vi "Detailed View.vi"(8 "error in (no error)":errorcluster, 10 "Server URL":refnum<k21>="\\\\localhost\\ABCDEFG", 11 "Client Message Queues":T1) -> ()   [LabVIEW 2024]
doc: "This VI is a user interface VI of the client and is used to display the detailed information of a subsystem, including the graphic subsystem view, alarm & event view, and historical data view."
uses:
  Shared/Message Queue/Client Message Queues.ctl
  Shared/Message Queue/Message Cluster.ctl
  Controls/Client/Detailed View - Data.ctl
  Error Handlers/Error Message.ctl
  Shared/Message Queue.lvlib
  Shared/User Event - Stop.lvlib
panel:
  in  "Exit":bool
  in  "Refresh":bool
  in  "Alarm & Event List":bool
  in  "Subsystem":string(combo)
  in  "Historical Trend":bool
  in  "Subsystem View":bool
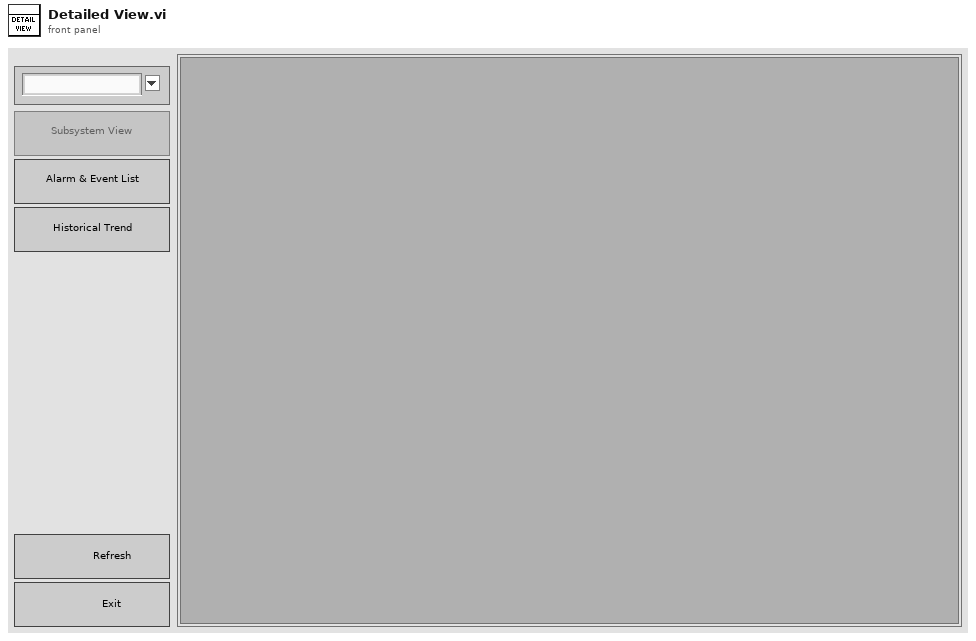
[diagram p1: front panel]
types:
  T1 = typedef "Message Queue.lvlib/Client Message Queues.ctl" = cluster{"Client Main":refnum<queue>, "Detailed View":refnum<queue>}
  T2 = typedef "Detailed View - Data.ctl" = cluster{"Current View Name":string, "Current View":refnum<vi>, "Current Subsystem":string, "Subview Reference Map":variant, "Subview Stop Events":refnum<user-event>[], "Detailed View Stop Event":refnum<user-event>, "Subview Switch Buttons Map":variant, "Client Message Queues":T1}
  T3 = typedef "Error Message.ctl" = cluster{"Error":errorcluster, "Component":string}
  T4 = enum8{"Enabled", "Disabled", "Disabled and Grayed Out"}
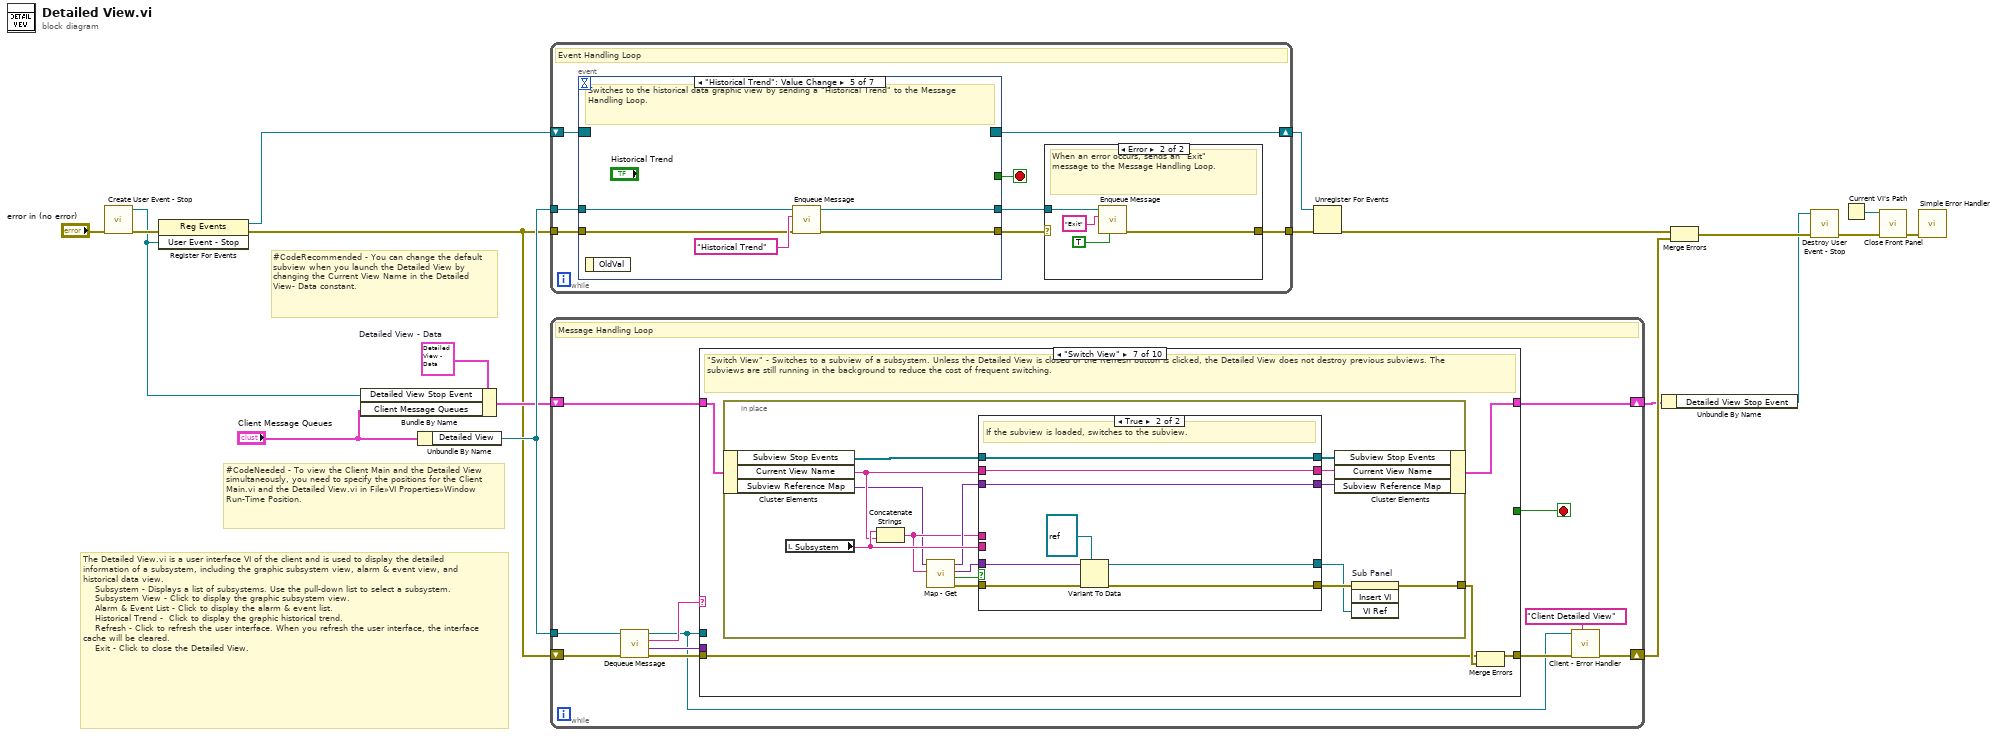
[diagram p0: block diagram]
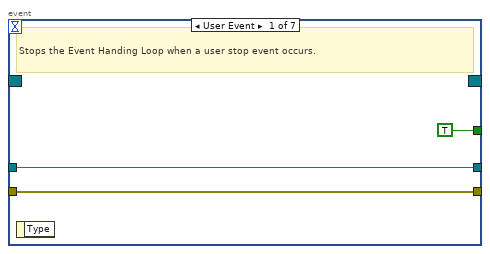
[diagram p3: hidden frame]
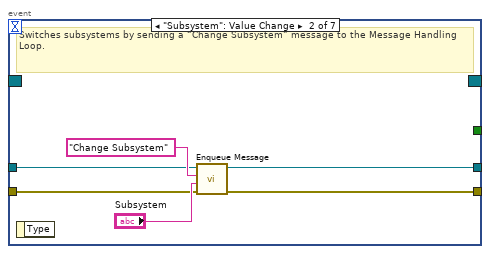
[diagram p4: hidden frame]
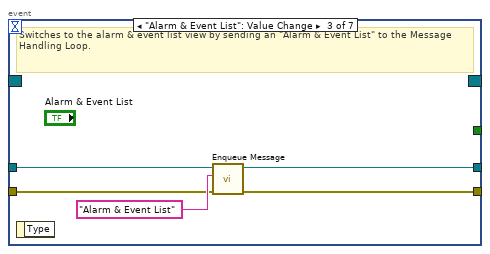
[diagram p5: hidden frame]
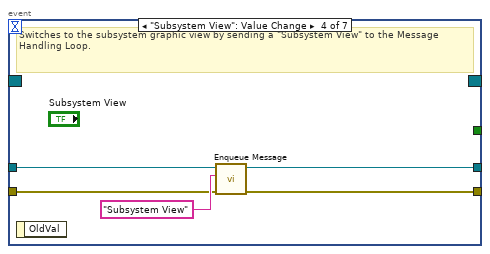
[diagram p6: hidden frame]
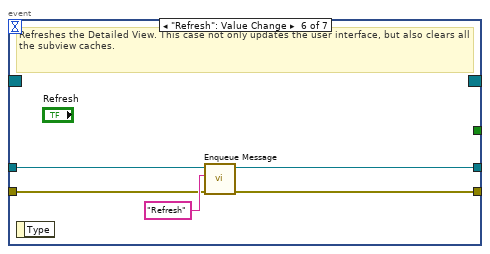
[diagram p7: hidden frame]
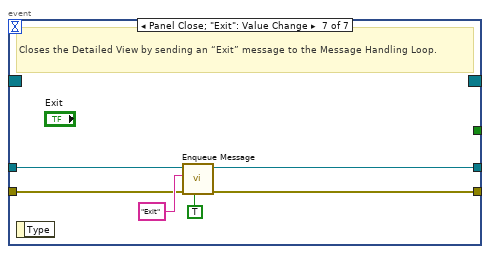
[diagram p8: hidden frame]
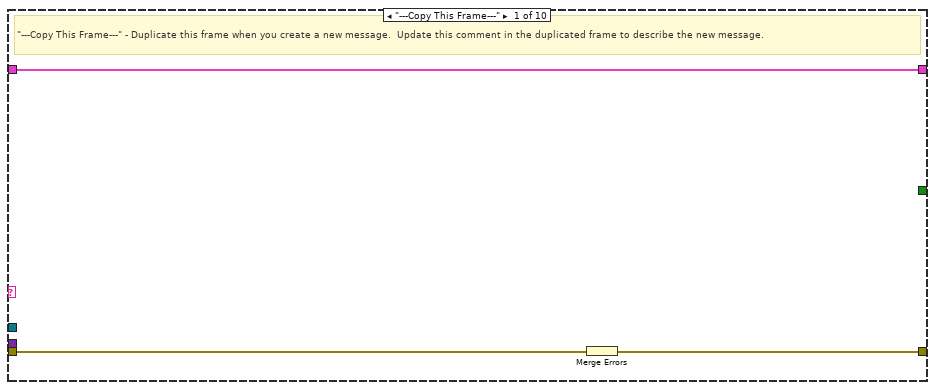
[diagram p9: hidden frame]
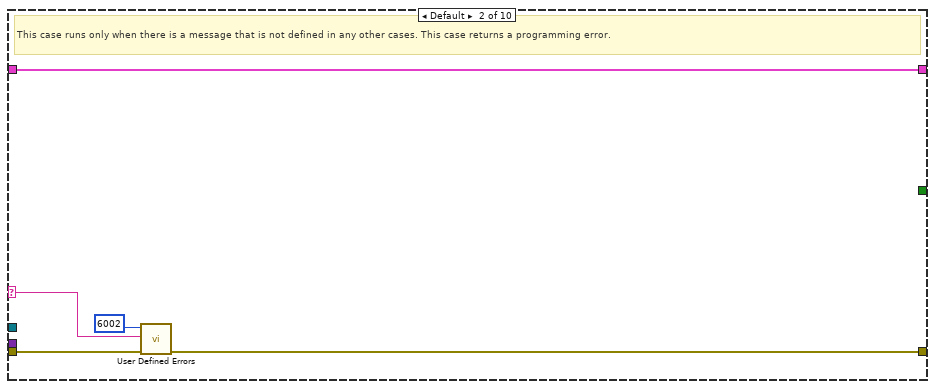
[diagram p10: hidden frame]
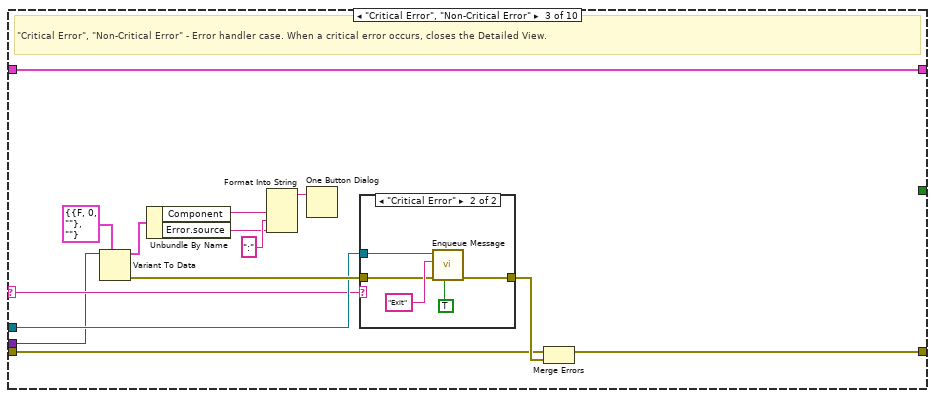
[diagram p11: hidden frame]
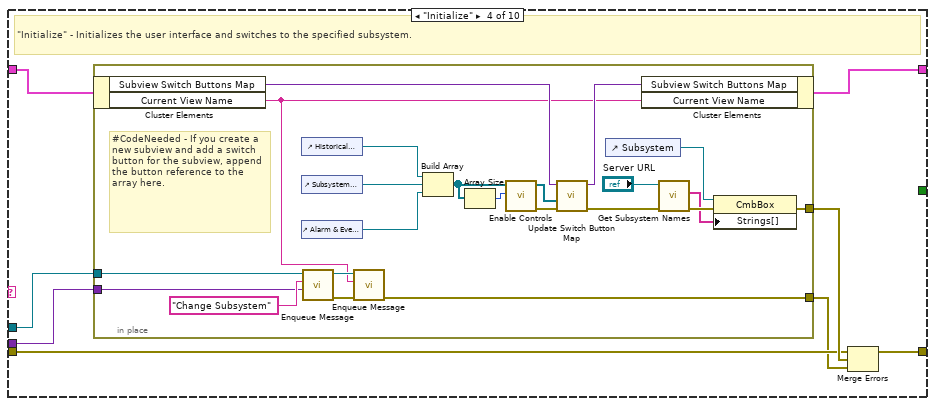
[diagram p13: hidden frame]
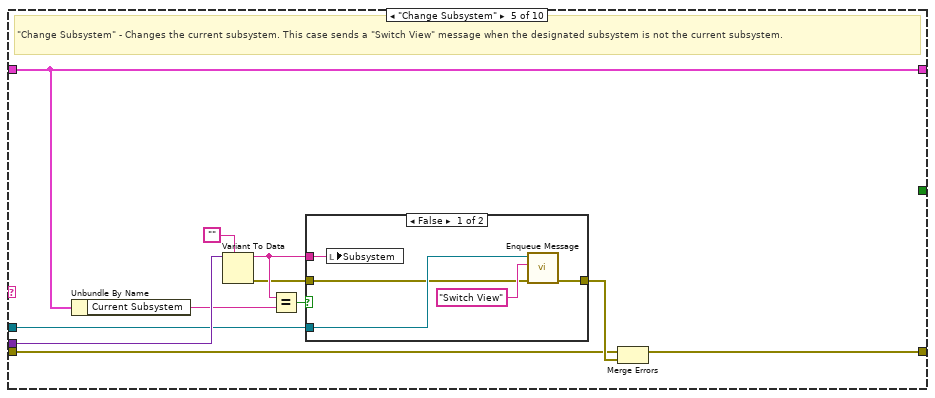
[diagram p14: hidden frame]
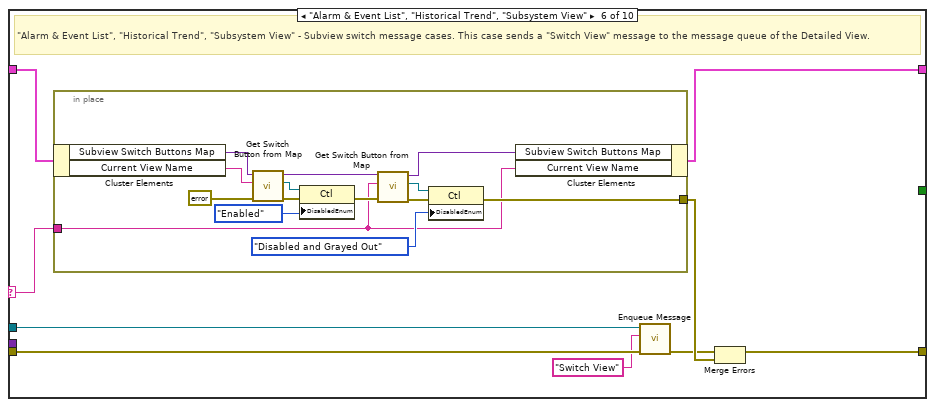
[diagram p16: hidden frame]
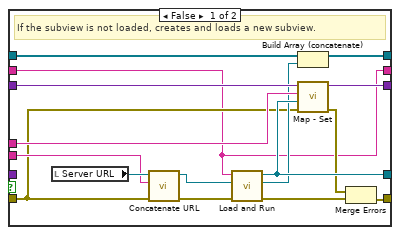
[diagram p17: hidden frame]
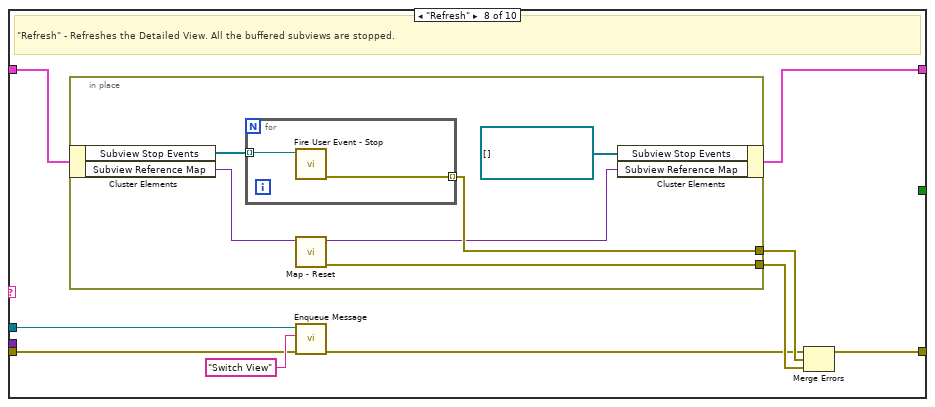
[diagram p18: hidden frame]
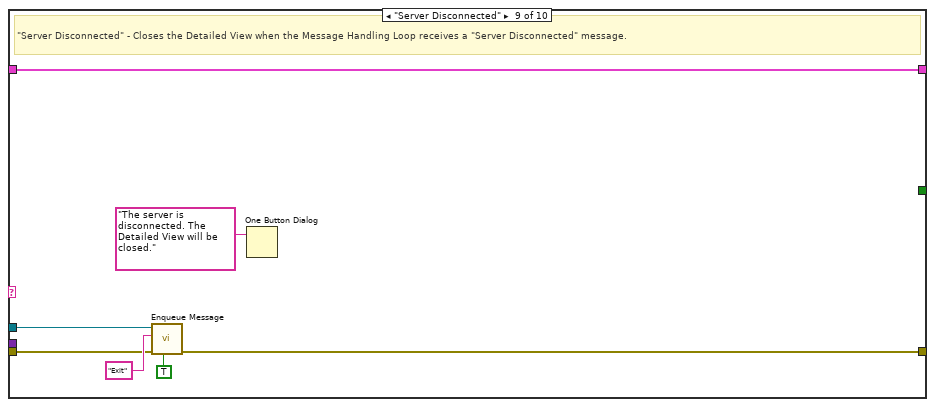
[diagram p19: hidden frame]
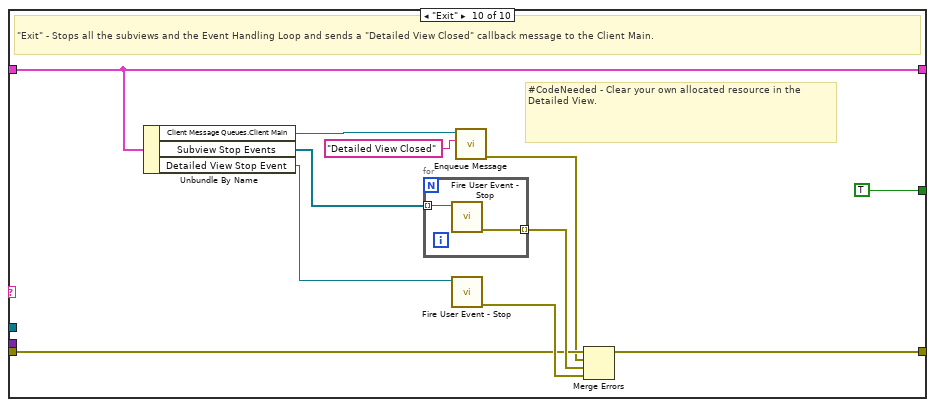
[diagram p20: hidden frame]
diagram:
  w12 = T2 {"Current View Name"="Subsystem View", "Current View"=refnum, "Current Subsystem"="", "Subview Reference Map"=variant, "Subview Stop Events"=[], "Detailed View Stop Event"=refnum, "Subview Switch Buttons Map"=variant, "Client Message Queues"={"Client Main"=refnum, "Detailed View"=refnum}}  # Detailed View - Data
  # "#CodeNeeded - To view the Client Main and the Detailed View simultaneously, you need to specify the positions for the Client Main.vi and the Detailed View.vi in File»VI Properties»Window Run-Time Position."
  # "#CodeRecommended - You can change the default subview when you launch the Detailed View by changing the Current View Name in the Detailed View- Data constant."
  # "The Detailed View.vi is a user interface VI of the client and is used to display the detailed information of a subsystem, including the graphic subsystem view, alarm & event view, and historical data view.\n    Subsystem - Displays a list of subsystems. Use the pull-down list to select a subsystem. \n    Subsystem View - Click to display the graphic subsystem view.\n    Alarm & Event List - Click to display the alarm & event list.\n    Historical Trend -  Click to display the graphic historical trend.\n    Refresh - Click to refresh the user interface. When you refresh the user interface, the interface cache will be cleared.\n    Exit - Click to close the Detailed View."
  n1 = call "Create User Event - Stop.vi"("error in (no error)"="error in (no error)") -> ("error out"=w4:errorcluster, "User Event - Stop"=w1:refnum<user-event>)  [unwired: 9 in]
  n2 = register-events(error in=w4, w1) -> (reference out=w2:refnum<event-registration>, error out=w3:errorcluster)  [unwired: 1 in]
  n3 = Bundle By Name(cluster=w12, "Detailed View Stop Event"=w1, "Client Message Queues"="Client Message Queues") -> (w6:T2)
  n4 = Unbundle By Name("Client Message Queues") -> ("Detailed View"=w13:refnum<queue>)
  n5 = while "Event Handling Loop" {
    tunnel: w13 -> [w27]
    tunnel: [w22] -> w16
    shift-right: [w23] -> w15
    shift-left: w2 -> [w24]
    tunnel: w3 -> [w20]
    stop <- w21 stop-if-true
    # "Event Handling Loop"
    n6 = event shown="[4] \"Historical Trend\": Value Change" {
      selector: w24 -> [_ _ _ _ _ _ _]
      dyn-events: [_ _ _ _ _ _ _] -> w23
      timeout: _ -> [_ _ _ _ _ _ _]
      tunnel: [TRUE ("Discard?") _ _ _ _ _ _] -> w21
      tunnel: w27 -> [w35 w40 w45 w50 w55 w61 w65]
      tunnel: [w33 w38 w43 w48 w53 w58 w63] -> w25
      tunnel: [w35 w39 w44 w49 w54 w60 w64] -> w26
      tunnel: w20 -> [w33 w36 w42 w47 w52 w57 w62]
      event User Event {
        # "Stops the Event Handing Loop when a user stop event occurs."
        n7 = event-data() -> ()  [unwired: 1 in, 1 out]
      }
      event "Subsystem": Value Change {
        # "Switches subsystems by sending a “Change Subsystem” message to the Message Handling Loop."
        n8 = event-data() -> ()  [unwired: 1 in, 1 out]
        n9 = call "Enqueue Message.vi"("error in (no error)"=w36, "Message Data"="Subsystem", "Message"="Change Subsystem", "Message Queue"=w40) -> ("error out"=w38:errorcluster, "dup Message Queue"=w39:refnum<queue>)  [unwired: 6 in]
      }
      event "Alarm & Event List": Value Change {
        # "Switches to the alarm & event list view by sending an \"Alarm & Event List\" to the Message Handling Loop."
        n10 = event-data() -> ()  [unwired: 1 in, 1 out]
        n11 = call "Enqueue Message.vi"("error in (no error)"=w42, "Message"="Alarm & Event List", "Message Queue"=w45) -> ("error out"=w43:errorcluster, "dup Message Queue"=w44:refnum<queue>)  [unwired: 7 in]
      }
      event "Subsystem View": Value Change {
        # "Switches to the subsystem graphic view by sending a \"Subsystem View\" to the Message Handling Loop."
        n12 = event-data() -> ()  [unwired: 1 in, 1 out]
        n13 = call "Enqueue Message.vi"("error in (no error)"=w47, "Message"="Subsystem View", "Message Queue"=w50) -> ("error out"=w48:errorcluster, "dup Message Queue"=w49:refnum<queue>)  [unwired: 7 in]
      }
      event "Historical Trend": Value Change {
        # "Switches to the historical data graphic view by sending a \"Historical Trend\" to the Message Handling Loop."
        n14 = event-data() -> ()  [unwired: 1 in, 1 out]
        n15 = call "Enqueue Message.vi"("error in (no error)"=w52, "Message"="Historical Trend", "Message Queue"=w55) -> ("error out"=w53:errorcluster, "dup Message Queue"=w54:refnum<queue>)  [unwired: 7 in]
      }
      event "Refresh": Value Change {
        # "Refreshes the Detailed View. This case not only updates the user interface, but also clears all the subview caches."
        n16 = event-data() -> ()  [unwired: 1 in, 1 out]
        n17 = call "Enqueue Message.vi"("error in (no error)"=w57, "Message"="Refresh", "Message Queue"=w61) -> ("error out"=w58:errorcluster, "dup Message Queue"=w60:refnum<queue>)  [unwired: 7 in]
      }
      event Panel Close; "Exit": Value Change {
        # "Closes the Detailed View by sending an “Exit” message to the Message Handling Loop."
        n18 = event-data() -> ()  [unwired: 1 in, 1 out]
        n19 = call "Enqueue Message.vi"("Priority Message? (F)"=TRUE, "error in (no error)"=w62, "Message"="Exit", "Message Queue"=w65) -> ("error out"=w63:errorcluster, "dup Message Queue"=w64:refnum<queue>)  [unwired: 6 in]
      }
    }
    n20 = case shown="Error" w25 {
      selector: w25 -> [w28 _]
      tunnel: w26 -> [_ w32]
      tunnel: [w28 w29] -> w22
      frame No Error {
      }
      frame Error {
        # "When an error occurs, sends an \"Exit\" message to the Message Handling Loop."
        n21 = call "Enqueue Message.vi"("Priority Message? (F)"=TRUE, "Message"="Exit", "Message Queue"=w32) -> ("error out"=w29:errorcluster)  [unwired: 7 in, 1 out]
      }
    }
  }
  n22 = while "Message Handling Loop" {
    tunnel: w13 -> [w72]
    shift-right: [w78] -> w11
    shift-left: w6 -> [w79]
    shift-right: [w70] -> w19
    shift-left: w3 -> [w76]
    stop <- w77 stop-if-true
    # "Message Handling Loop"
    n23 = call "Dequeue Message.vi"("error in (no error)"=w76, "Message Queue"=w72) -> ("error out"=w75:errorcluster, "Message Data"=w73:variant, "Message"=w74:string, "dup Message Queue"=w69:refnum<queue>)  [unwired: 6 in]
    n24 = case "Message Cases" shown="\"Switch View\"" w74 {
      selector: w74 -> [_ w84 w96 _ _ w157 _ _ _ _]
      tunnel: w69 -> [_ _ w97 w110 w144 w163 _ w227 w241 _]
      tunnel: w75 -> [w82 w83 w88 w113 w138 w162 w178 w228 w242 w249]
      tunnel: [w81 w85 w95 w115 w148 w160 w182 w230 w240 w255] -> w71
      tunnel: w79 -> [w80 w87 w101 w112 w142 w159 w179 w224 w245 w253]
      tunnel: [w80 w87 w101 w111 w142 w158 w180 w223 w245 w253] -> w78
      tunnel: [_ _ _ _ _ _ _ _ _ TRUE] -> w77
      tunnel: w73 -> [_ _ w94 w109 w147 _ _ _ _ _]
      frame "---Copy This Frame---" {
        # "\"---Copy This Frame---\" - Duplicate this frame when you create a new message.  Update this comment in the duplicated frame to describe the new message."
        n25 = Merge Errors(w82) -> (w81:errorcluster)
      }
      frame Default {
        # "This case runs only when there is a message that is not defined in any other cases. This case returns a programming error."
        n26 = call "User Defined Errors.vi"("error in (no error)"=w83, "Parameter 1"=w84, "Error Code (0)"=6002 ("error code (0)")) -> ("error out"=w85:errorcluster)  [unwired: 8 in]
      }
      frame "Critical Error", "Non-Critical Error" {
        # "\"Critical Error\", \"Non-Critical Error\" - Error handler case. When a critical error occurs, closes the Detailed View."
        n27 = Variant To Data(type=T3 {"Error"={"status"=FALSE, "code"=0, "source"=""}, "Component"=""} ("Error Message"), Variant=w94) -> (data=w100:T3, error out=w99:errorcluster)  [unwired: 1 in]
        n28 = Unbundle By Name(w100) -> ("Component"=w93:string, "Error.source"=w91:string)
        n29 = Format Into String(w93, ":" ("input 1"), w91) -> (resulting string=w90:string)  [unwired: 3 in, 1 out]
        n30 = One Button Dialog(message=w90) -> ()  [unwired: 1 in, 1 out]
        n31 = case shown="\"Critical Error\"" w96 {
          tunnel: [w102 w105] -> w89
          tunnel: w97 -> [_ w104]
          tunnel: w99 -> [w102 w103]
          frame Default {
          }
          frame "Critical Error" {
            n32 = call "Enqueue Message.vi"("Priority Message? (F)"=TRUE, "error in (no error)"=w103, "Message"="Exit", "Message Queue"=w104) -> ("error out"=w105:errorcluster)  [unwired: 6 in, 1 out]
          }
        }
        n33 = Merge Errors(w88, w89) -> (w95:errorcluster)
      }
      frame "Initialize" {
        # "\"Initialize\" - Initializes the user interface and switches to the specified subsystem."
        n34 = in-place {
          in-place-border: [w135] -> w114
          in-place-border: w110 -> [w119]
          in-place-border: w109 -> [w118]
          in-place-border: [w117] -> w108
          # "#CodeNeeded - If you create a new subview and add a switch button for the subview, append the button reference to the array here."
          n35 = in-place-cluster #1(w112) -> ("Subview Switch Buttons Map"=w124:variant, "Current View Name"=w116:string)
          n36 = control-ref of="Historical Trend"() -> (w134:refnum<vi>)
          n37 = control-ref of="Subsystem View"() -> (w133:refnum<vi>)
          n38 = control-ref of="Alarm & Event List"() -> (w131:refnum<vi>)
          n39 = call "Enqueue Message.vi"("Message Data"=w118, "Message"="Change Subsystem", "Message Queue"=w119) -> ("error out"=w122:errorcluster, "dup Message Queue"=w121:refnum<queue>)  [unwired: 7 in]
          n40 = call "Enqueue Message.vi"("error in (no error)"=w122, "Message"=w116, "Message Queue"=w121) -> ("error out"=w117:errorcluster)  [unwired: 7 in, 1 out]
          n41 = Build Array(w134, w133, w131) -> (w127:refnum<vi>[])
          n42 = Array Size(array=w127) -> (size(s)=w126:i32)
          n43 = call "Enable Controls.vi"("Number of Enabled Controls"=w126, "Controls"=w127) -> ("error out"=w129:errorcluster, "dup Controls"=w128:refnum<vi>[])  [unwired: 8 in]
          n44 = call "Update Switch Button Map.vi"("error in (no error)"=w129, "Binding Control Refnums"=w128, "URL Refnum Map In"=w124) -> ("error out"=w132:errorcluster, "URL Refnum Map Out"=w123:variant)  [unwired: 7 in]
          n45 = control-ref of="Subsystem"() -> (w130:refnum<vi>)
          n46 = in-place-cluster #1("Subview Switch Buttons Map"=w123, "Current View Name"=w116) -> (w111:T2)
          n47 = call "Get Subsystem Names.vi"("error in (no error)"=w132, "Server URL"="Server URL") -> ("error out"=w137:errorcluster, "Subsystem Names"=w125:string[])  [unwired: 7 in, 1 out]
          n48 = property class="CmbBox"(reference=w130, error in=w137, "Strings[]"=w125) -> (error out=w135:errorcluster)  [unwired: 1 out]
        }
        n49 = Merge Errors(w113, w114, w108) -> (w115:errorcluster)
      }
      frame "Change Subsystem" {
        # "\"Change Subsystem\" - Changes the current subsystem. This case sends a \"Switch View\" message when the designated subsystem is not the current subsystem."
        n50 = Unbundle By Name(w142) -> ("Current Subsystem"=w141:string)
        n51 = Variant To Data(type="" ("Value (Signaling)"), Variant=w147) -> (data=w143:string, error out=w140:errorcluster)  [unwired: 1 in]
        n52 = Equal?(x=w143, y=w141) -> (x = y?=w145:bool)
        n53 = case shown="False" w145 {
          tunnel: w143 -> [w151 _]
          tunnel: w144 -> [w153 _]
          tunnel: w140 -> [w150 w154]
          tunnel: [w149 w154] -> w139
          frame False {
            n54 = local write "Subsystem"(w151) -> ()
            n55 = call "Enqueue Message.vi"("error in (no error)"=w150, "Message"="Switch View", "Message Queue"=w153) -> ("error out"=w149:errorcluster)  [unwired: 7 in, 1 out]
          }
          frame True {
          }
        }
        n56 = Merge Errors(w138, w139) -> (w148:errorcluster)
      }
      frame "Alarm & Event List", "Historical Trend", "Subsystem View" {
        # "\"Alarm & Event List\", \"Historical Trend\", \"Subsystem View\" - Subview switch message cases. This case sends a \"Switch View\" message to the message queue of the Detailed View."
        n57 = in-place {
          in-place-border: w157 -> [w165]
          in-place-border: [w168] -> w156
          n58 = in-place-cluster #2(w159) -> ("Subview Switch Buttons Map"=w177:variant, "Current View Name"=w176:string)
          n59 = call "Get Switch Button from Map.vi"("error in (no error)"=errorcluster {"status"=FALSE, "code"=0, "source"=""} ("error out"), "Subview Command"=w176, "URL Refnum Map"=w177) -> ("error out"=w175:errorcluster, "Switch Button Refnum"=w174:refnum<vi>, "dup URL Refnum Map"=w170:variant)  [unwired: 5 in, 1 out]
          n60 = property class="Ctl"(reference=w174, error in=w175, "DisabledEnum"=T4."Enabled" ("Disabled")) -> (error out=w173:errorcluster)  [unwired: 1 out]
          n61 = call "Get Switch Button from Map.vi"("error in (no error)"=w173, "Subview Command"=w165, "URL Refnum Map"=w170) -> ("error out"=w171:errorcluster, "Switch Button Refnum"=w172:refnum<vi>, "dup URL Refnum Map"=w169:variant)  [unwired: 5 in, 1 out]
          n62 = property class="Ctl"(reference=w172, error in=w171, "DisabledEnum"=T4."Disabled and Grayed Out" ("Disabled")) -> (error out=w168:errorcluster)  [unwired: 1 out]
          n63 = in-place-cluster #2("Subview Switch Buttons Map"=w169, "Current View Name"=w165) -> (w158:T2)
        }
        n64 = call "Enqueue Message.vi"("error in (no error)"=w162, "Message"="Switch View", "Message Queue"=w163) -> ("error out"=w155:errorcluster)  [unwired: 7 in, 1 out]
        n65 = Merge Errors(w155, w156) -> (w160:errorcluster)
      }
      frame "Switch View" {
        # "\"Switch View\" - Switches to a subview of a subsystem. Unless the Detailed View is closed or the Refresh button is clicked, the Detailed View does not destroy previous subviews. The subviews are still running in the background to reduce the cost of frequent switching."
        n66 = in-place {
          in-place-border: [w183] -> w181
          n67 = in-place-cluster #3(w179) -> ("Subview Stop Events"=w188:refnum<user-event>[], "Current View Name"=w187:string, "Subview Reference Map"=w186:variant)
          n68 = local read "Subsystem"() -> (w196:string)
          n69 = Concatenate Strings(w196, w187) -> (w192:string)
          n70 = call "Map - Get.vi"("Key"=w192, "Map In"=w186) -> ("error out"=w197:errorcluster, "Found?"=w185:bool, "Value"=w184:variant, "Map Out"=w193:variant)  [unwired: 6 in]
          n71 = case shown="True" w185 {
            tunnel: w188 -> [w213 w217]
            tunnel: w196 -> [w207 _]
            tunnel: w187 -> [w198 w214]
            tunnel: [w202 w218] -> w195
            tunnel: [w211 w219] -> w194
            tunnel: w184 -> [_ w221]
            tunnel: w193 -> [w210 w216]
            tunnel: w192 -> [w209 _]
            tunnel: [w208 w216] -> w191
            tunnel: [w198 w214] -> w190
            tunnel: [w206 w217] -> w189
            tunnel: w197 -> [w199 w215]
            frame False {
              # "If the subview is not loaded, creates and loads a new subview."
              n72 = local read "Server URL"() -> (w212:refnum<k21>)
              n73 = call "Concatenate URL.vi"("error in (no error)"=w199, "Child Name"=w207, "Parent URL"=w212) -> ("error out"=w204:errorcluster, "Child URL"=w205:refnum<k21>)  [unwired: 7 in]
              n74 = call "Load and Run.vi"("error in (no error)"=w204, "Subsystem URL"=w205, "Subview"=w198) -> ("error out"=w201:errorcluster, "Current Stop Event"=w203:refnum<user-event>, "Subview VI Reference"=w211:refnum<vi>)  [unwired: 6 in]
              n75 = Build Array (concatenate)(w213, w203) -> (w206:refnum<user-event>[])
              n76 = call "Map - Set.vi"("error in (no error)"=w199, "Value"=w211, "Key"=w209, "Map In"=w210) -> ("error out"=w200:errorcluster, "Map Out"=w208:variant)  [unwired: 5 in, 1 out]
              n77 = Merge Errors(w200, w201) -> (w202:errorcluster)
            }
            frame True {
              # "If the subview is loaded, switches to the subview."
              n78 = Variant To Data(error in=w215, type=refnum<vi> refnum ("vi refnum out"), Variant=w221) -> (data=w219:refnum<vi>, error out=w218:errorcluster)
            }
          }
          n79 = in-place-cluster #3("Subview Stop Events"=w189, "Current View Name"=w190, "Subview Reference Map"=w191) -> (w180:T2)
          n80 = invoke on="Sub Panel" class="SubPnl" method="Insert VI"(error in=w195, "VI Ref"=w194) -> (error out=w183:errorcluster)  [unwired: 2 in, 3 out]
        }
        n81 = Merge Errors(w178, w181) -> (w182:errorcluster)
      }
      frame "Refresh" {
        # "\"Refresh\" - Refreshes the Detailed View. All the buffered subviews are stopped."
        n82 = in-place {
          in-place-border: [w236] -> w226
          in-place-border: [w235] -> w225
          n83 = in-place-cluster #4(w224) -> ("Subview Stop Events"=w231:refnum<user-event>[], "Subview Reference Map"=w234:variant)
          n84 = for {
            tunnel: [w238] -> w235 mode=indexing
            tunnel: w231 -> [w237] mode=indexing
            n85 = call "Fire User Event - Stop.vi"("User Event - Stop"=w237) -> ("error out"=w238:errorcluster)  [unwired: 10 in]
          }
          n86 = call "Map - Reset.vi"("Map In"=w234) -> ("error out"=w236:errorcluster, "Map Out"=w233:variant)  [unwired: 9 in]
          n87 = in-place-cluster #4("Subview Stop Events"=refnum<user-event>[] [], "Subview Reference Map"=w233) -> (w223:T2)
        }
        n88 = call "Enqueue Message.vi"("error in (no error)"=w228, "Message"="Switch View", "Message Queue"=w227) -> ("error out"=w222:errorcluster)  [unwired: 7 in, 1 out]
        n89 = Merge Errors(w222, w225, w226) -> (w230:errorcluster)
      }
      frame "Server Disconnected" {
        # "\"Server Disconnected\" - Closes the Detailed View when the Message Handling Loop receives a \"Server Disconnected\" message."
        n90 = call "Enqueue Message.vi"("Priority Message? (F)"=TRUE, "error in (no error)"=w242, "Message"="Exit", "Message Queue"=w241) -> ("error out"=w240:errorcluster)  [unwired: 6 in, 1 out]
        n91 = One Button Dialog(message="The server is disconnected. The Detailed View will be closed.") -> ()  [unwired: 1 in, 1 out]
      }
      frame "Exit" {
        # "#CodeNeeded - Clear your own allocated resource in the Detailed View."
        # "\"Exit\" - Stops all the subviews and the Event Handling Loop and sends a \"Detailed View Closed\" callback message to the Client Main."
        n92 = Unbundle By Name(w253) -> ("Client Message Queues.Client Main"=w248:refnum<queue>, "Subview Stop Events"=w251:refnum<user-event>[], "Detailed View Stop Event"=w250:refnum<user-event>)
        n93 = for {
          tunnel: [w258] -> w252 mode=indexing
          tunnel: w251 -> [w257] mode=indexing
          n94 = call "Fire User Event - Stop.vi"("User Event - Stop"=w257) -> ("error out"=w258:errorcluster)  [unwired: 10 in]
        }
        n95 = call "Fire User Event - Stop.vi"("User Event - Stop"=w250) -> ("error out"=w254:errorcluster)  [unwired: 10 in]
        n96 = call "Enqueue Message.vi"("Message"="Detailed View Closed", "Message Queue"=w248) -> ("error out"=w247:errorcluster)  [unwired: 8 in, 1 out]
        n97 = Merge Errors(w249, w247, w252, w254) -> (w255:errorcluster)
      }
    }
    n98 = call "Client - Error Handler.vi"("Component"="Client Detailed View", "error in (no error)"=w71, "Message Queue"=w69) -> ("error out"=w70:errorcluster)  [unwired: 8 in]
  }
  n99 = Unregister For Events(event registration refnum=w15, error in=w16) -> (error out=w17:errorcluster)
  n100 = Unbundle By Name(w11) -> ("Detailed View Stop Event"=w10:refnum<user-event>)
  n101 = Merge Errors(w17, w19) -> (w18:errorcluster)
  n102 = call "Destroy User Event - Stop.vi"("error in (no error)"=w18, "User Event - Stop"=w10) -> ("error out"=w8:errorcluster)  [unwired: 9 in]
  n103 = Current VI's Path() -> (path=w9:path)
  n104 = call "Close Front Panel.vi"("error in (no error)"=w8, "VI File Path"=w9) -> ("error out"=w7:errorcluster)  [unwired: 9 in]
  n105 = call <vilib>:"Simple Error Handler.vi"("error in (no error)"=w7) -> ()  [unwired: 4 in, 5 out]
